vi "Print Best Solution To Front Panel.vi"(8 "error in (no error)":errorcluster, 10 "OSSP_Problem in":refnum<class "OSSP_Problem.lvclass">, 11 "GA.lvclass":refnum<class "GA.lvclass">) -> (0 "error out":errorcluster, 1 "Result":u16, 2 "String":string, 3 "GA out":refnum<class "GA.lvclass">)   [LabVIEW 2013]
uses:
  Classes/GA.lvclass
  Classes/OSSP_Problem.lvclass
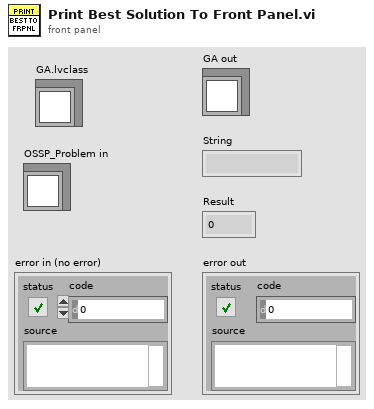
[diagram p1: front panel]
types:
  T1 = typedef "Solution_GA.ctl" = cluster{"Schedule":u16[], "Fitness":u16, "Fitness Valid?":bool}
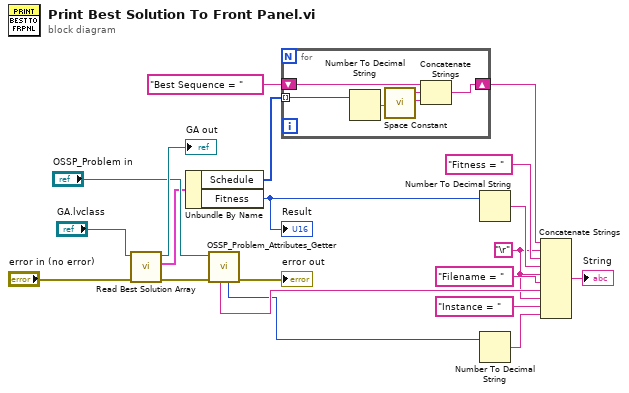
[diagram p0: block diagram]
diagram:
  w2 = "\r"
  n1 = call-dynamic "Read Best Solution Array.vi"("error in (no error)"="error in (no error)", "GA in"="GA.lvclass") -> ("error out"=w3:errorcluster, "Best Solution"=w4:T1, "GA out"=→"GA out":refnum<class "GA.lvclass">)  [unwired: 7 in]
  n2 = Unbundle By Name(w4) -> ("Schedule"=w5:u16[], "Fitness"=w1:u16)
  "Result" <- w1
  n3 = call "OSSP_Problem_Attributes_Getter.vi"("error in (no error)"=w3, "OSSP_Problem in"="OSSP_Problem in") -> ("error out"=→"error out":errorcluster, "Instance"=w7:u8, "Filename"=w9:string)  [unwired: 3 in, 4 out]
  n4 = for {
    tunnel: w5 -> [w25] mode=indexing
    shift-right: [w21] -> w13
    shift-left: "Best Sequence = " -> [w24]
    n5 = Number To Decimal String(number=w25) -> (decimal integer string=w23:string)  [unwired: 1 in]
    n6 = call <vilib>:"Space Constant.vi"() -> ("String"=w22:string)
    n7 = Concatenate Strings(w24, w23, w22) -> (w21:string)
  }
  n8 = Number To Decimal String(number=w1) -> (decimal integer string=w12:string)  [unwired: 1 in]
  n9 = Number To Decimal String(number=w7) -> (decimal integer string=w6:string)  [unwired: 1 in]
  n10 = Concatenate Strings(w13, w2, "Fitness = " ("string"), w12, w2, "Filename = " ("string"), w9, w2, "Instance = " ("string"), w6) -> (→"String":string)
